vi "CleanUpNode.vi"(8 "error in (no error)":errorcluster, 10 "Parameters":variant, 11 "CI Project in":refnum<class "CI Project.lvclass">) -> (0 "error out":errorcluster, 3 "CI Project out":refnum<class "CI Project.lvclass">)   [LabVIEW 2014, in "CI Project.lvclass"]
doc: "This VI will clean any reference handled internally in the node"
uses:
  CI Project.lvclass
  <vilib>/ni/Configuration Framework/Node/NISE_CEF_Node.lvclass/NISE_CEF_Node.ctl
  <vilib>/ni/Configuration Framework/Node/NISE_CEF_Node.lvclass
  <vilib>/ni/Configuration Framework/Node/ReadChildren.vi
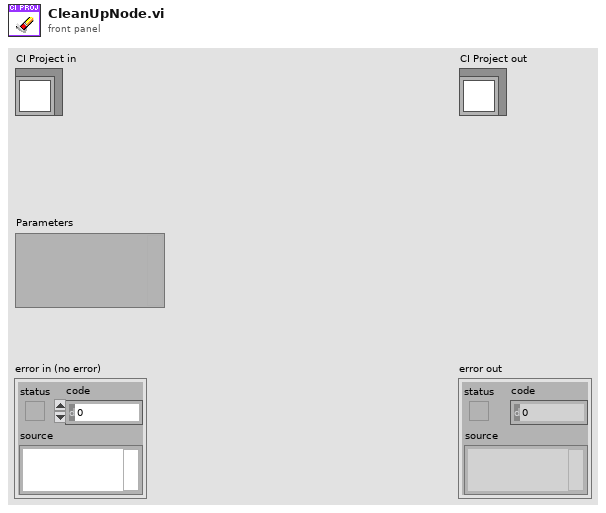
[diagram p1: front panel]
types:
  T1 = typedef "NISE_CEF_Node.lvclass/NodeRef.ctl" = refnum<data-value>
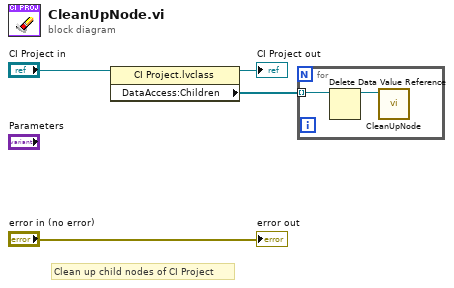
[diagram p0: block diagram]
diagram:
  # "Clean up child nodes of CI Project"
  n1 = property class="CI Project.lvclass"(reference="CI Project in") -> (reference out=→"CI Project out":refnum<class "CI Project.lvclass">, "DataAccess:Children"=w4:T1[])  [unwired: 1 in, 1 out]
  n2 = for {
    tunnel: w4 -> [w5] mode=indexing
    n3 = Delete Data Value Reference(data value reference=w5) -> (data value=w6:refnum<class "NISE_CEF_Node.lvclass">)  [unwired: 1 in, 1 out]
    n4 = call-dynamic "CleanUpNode.vi"("NISE_CEF_Node in"=w6) -> ()  [unwired: 9 in, 2 out]
  }
  "error out" <- "error in (no error)"
